vi "SetPostProcessing.vi"(6 "Post Processing":refnum<vi>, 9 "Value":refnum<vi>, 10 "PpIndex":refnum<k24>, 11 ".NET Refnum in":refnum<k24>) -> ()   [LabVIEW 2018]
uses:
  D:/SVN/PM/sdk/AppSamples/LabVIEWSamples/trunk/Release/2018/Dependencies/PVCamNET.dll
  Dependencies/PVCamNET.dll
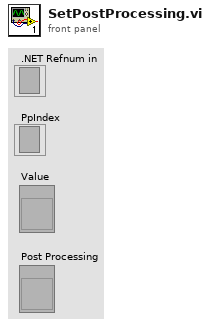
[diagram p1: front panel]
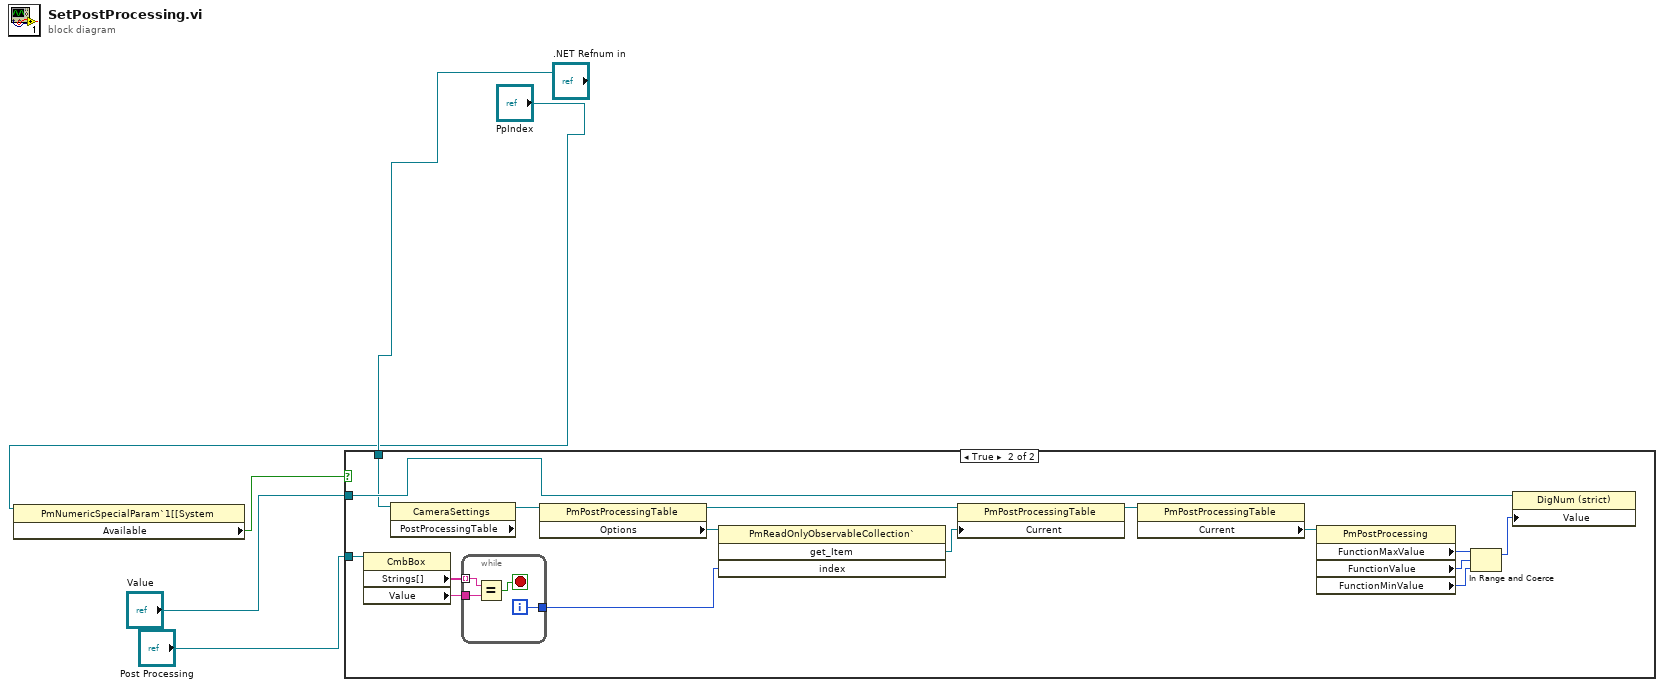
[diagram p0: block diagram]
diagram:
  n1 = property class="PmNumericSpecialParam`1[[System"(reference="PpIndex") -> ("Available"=w1:bool)  [unwired: 1 in, 2 out]
  n2 = case shown="True" w1 {
    tunnel: "Post Processing" -> [_ w16]
    tunnel: "Value" -> [_ w12]
    tunnel: ".NET Refnum in" -> [_ w7]
    frame False {
    }
    frame True {
      n3 = property class="CmbBox"(reference=w16) -> ("Strings[]"=w21:string[], "Value"=w20:string)  [unwired: 1 in, 2 out]
      n4 = property class="CameraSettings"(reference=w7) -> ("PostProcessingTable"=w6:refnum<k24>)  [unwired: 1 in, 2 out]
      n5 = while {
        tunnel: w21 -> [w25] mode=indexing
        tunnel: w20 -> [w24]
        tunnel: [w22] -> w14
        i -> [w22]
        stop <- w23 stop-if-true
        n6 = Equal?(x=w25, y=w24) -> (x = y?=w23:bool)
      }
      n7 = property class="PmPostProcessingTable"(reference=w6) -> (reference out=w19:refnum<k24>, "Options"=w15:refnum<k24>)  [unwired: 1 in, 1 out]
      n8 = invoke class="PmReadOnlyObservableCollection`" method="get_Item"(reference=w15, "index"=w14) -> ("get_Item"=w13:refnum<k24>)  [unwired: 2 in, 3 out]
      n9 = property class="PmPostProcessingTable"(reference=w19, "Current"=w13) -> (reference out=w18:refnum<k24>)  [unwired: 1 in, 1 out]
      n10 = property class="PmPostProcessingTable"(reference=w18) -> ("Current"=w17:refnum<k24>)  [unwired: 1 in, 2 out]
      n11 = property class="PmPostProcessing"(reference=w17) -> ("FunctionMaxValue"=w10:i32, "FunctionValue"=w9:i32, "FunctionMinValue"=w8:i32)  [unwired: 1 in, 2 out]
      n12 = In Range and Coerce(upper limit=w10, x=w9, lower limit=w8) -> (coerced(x)=w11:i32)  [unwired: 1 out]
      n13 = property class="DigNum (strict)"(reference=w12, "Value"=w11) -> ()  [unwired: 1 in, 2 out]
    }
  }
